vi "Area.vi"(8 "error in (no error)":errorcluster, 11 "IDrawable in":refnum<class "IDrawable.lvclass">) -> (0 "error out":errorcluster, 2 "Area":T1, 3 "IDrawable out":refnum<class "IDrawable.lvclass">)   [LabVIEW 2021, in "Picture2D.lvlib" / "IDrawable.lvclass"]
uses:
  IDrawable.lvclass
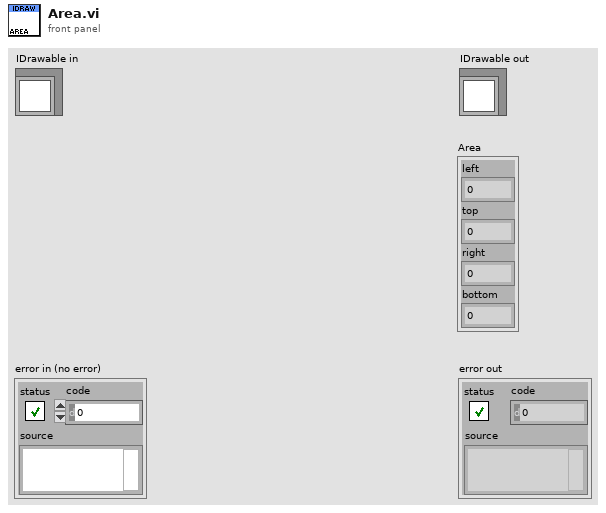
[diagram p1: front panel]
types:
  T1 = cluster{"left":i16, "top":i16, "right":i16, "bottom":i16}
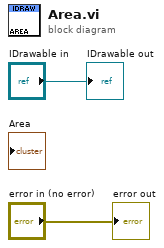
[diagram p0: block diagram]
diagram:
  "error out" <- "error in (no error)"
  "IDrawable out" <- "IDrawable in"
